vi "writeToXML.vi"(8 "error in (no error)":errorcluster, 10 "ClassLabel":string, 11 "MccRotTrack in":refnum<class "MccRotTrack.lvclass">) -> (0 "error out":errorcluster, 2 "XMLout":string, 3 "MccRotTrack out":refnum<class "MccRotTrack.lvclass">)   [LabVIEW 2022 SP3, in "TCSDataDefinitions.lvlib" / "TCSMountControlCommand.lvlib" / "CommandsForRotatorAxis.lvlib" / "MccRotTrack.lvclass"]
uses:
  MccRotTrack.lvclass
  MccRotTrack.lvclass/MccRotTrack.ctl
  CommandsForRotatorAxis.lvclass
  <userlib>/Common/XML/XMLGenerator/XMLGenerator.lvclass
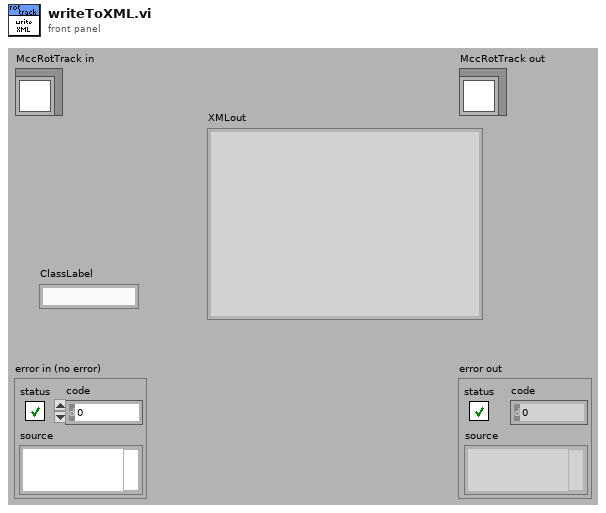
[diagram p1: front panel]
types:
  T1 = typedef "TCSDataDefinitions.lvlib/TCSMountControlCommand.lvlib/MountTrackStates.ctl" = enum16{"On", "Off"}
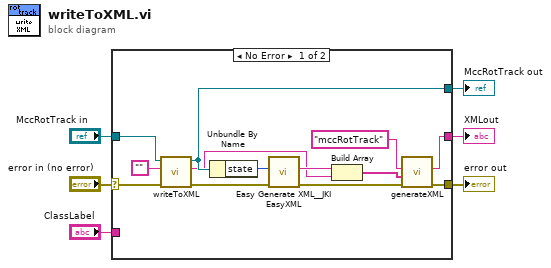
[diagram p0: block diagram]
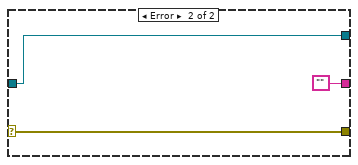
[diagram p2: hidden frame]
diagram:
  n1 = case shown="No Error" "error in (no error)" {
    selector: "error in (no error)" -> [w8 w22]
    tunnel: [w7 w22] -> w5
    tunnel: [w17 w21] -> w3
    tunnel: "MccRotTrack in" -> [w18 w21]
    tunnel: [w9 ""] -> w2
    tunnel: "ClassLabel" -> [_ _]
    frame No Error {
      n2 = call-parent "writeToXML.vi"("error in (no error)"=w8, "ClassLabel"="", "CommandsForRotatorAxis in"=w18) -> ("error out"=w15:errorcluster, "XMLout"=w13:string, "CommandsForRotatorAxis out"=w17:refnum<class "MccRotTrack.lvclass">)  [unwired: 6 in]
      n3 = Unbundle By Name(w17) -> ("state"=w16:T1)
      n4 = call <vilib>:"Easy Generate XML__JKI EasyXML.vi"("error in (no error)"=w15, "LabVIEW Data"=w16) -> ("error out"=w11:errorcluster, "XML String"=w14:string)  [unwired: 8 in]
      n5 = Build Array(w14, w13) -> (w12:string[])
      n6 = call <userlib>:"generateXML.vi"("error in"=w11, "childrenXML"=w12, "elementName"="mccRotTrack" ("Class Label")) -> ("error out"=w7:errorcluster, "XML out"=w9:string)  [unwired: 6 in, 1 out]
    }
    frame Error {
    }
  }
  "error out" <- w5
  "MccRotTrack out" <- w3
  "XMLout" <- w2
